vi "Number_to_string.vi"() -> ()   [LabVIEW 2019]
panel:
  out "decimal integer string":string
  out "Engineering string":string
  out "E-format string":string
  out "F-format string":string
  out "octal integer string":string
  out "hex integer string":string
  in  "precision":i16
  in  "number 2":dbl
  in  "width (-)":i16
  in  "number 1":i32
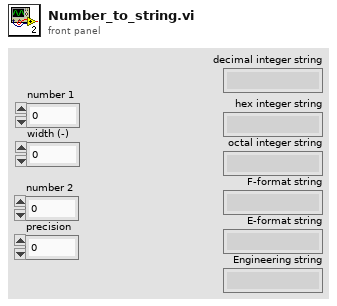
[diagram p1: front panel]
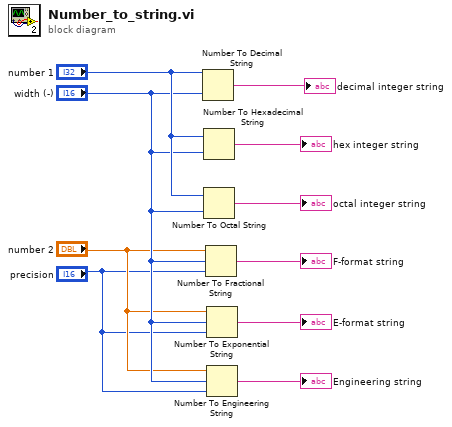
[diagram p0: block diagram]
diagram:
  n1 = Number To Decimal String(number="number 1", width (-)="width (-)") -> (decimal integer string=→"decimal integer string":string)
  n2 = Number To Hexadecimal String(1:"width (-)", 2:"number 1") -> (0:→"hex integer string":string)
  n3 = Number To Octal String(1:"width (-)", 2:"number 1") -> (0:→"octal integer string":string)
  n4 = Number To Fractional String(number="number 2", width (-)="width (-)", precision (6)="precision") -> (F-format string=→"F-format string":string)  [unwired: 1 in]
  n5 = Number To Exponential String(number="number 2", precision (6)="precision", 3:"width (-)") -> (E-format string=→"E-format string":string)  [unwired: 1 in]
  n6 = Number To Engineering String(2:"precision", 3:"width (-)", 4:"number 2") -> (0:→"Engineering string":string)  [unwired: 1 in]
